vi "GetGrabberPosition.vi"(8 "error in (no error)":errorcluster, 11 "JKI.Robot.SMO.Base.lvclass":refnum<class "JKI.Robot.SMO.Base.lvclass">) -> (0 "error out":errorcluster, 2 "SetGrabberPosition":dbl, 3 "JKI.Robot.SMO.Base.lvclass":refnum<class "JKI.Robot.SMO.Base.lvclass">)   [LabVIEW 2014, in "JKI.Robot.SMO.Base.lvclass"]
doc: "---------------------------------------------------------------\nJKI State Machine Objects™\nhttp://jki.net/state-machine-objects/\nCopyright (C) 2005-2015, JKI <info@jki.net>\nALL RIGHTS RESERVEDJKI State Machine Objects (SMO) 1.0.0.4\nJKI - JKI\nCopyright (c) 2015, JKI"
uses:
  JKI.Robot.SMO.Base.lvclass
panel:
  # "For instructions on how to use the JKI State Machine Objects, examples and video tutorials, visit:\nhttp://jki.net/state-machine-objects/\n\nJKI State Machine Objects™\nhttp://jki.net/state-machine-objects/\nCopyright (C) 2005-2015, JKI <info@jki.net>\nALL RIGHTS RESERVED"
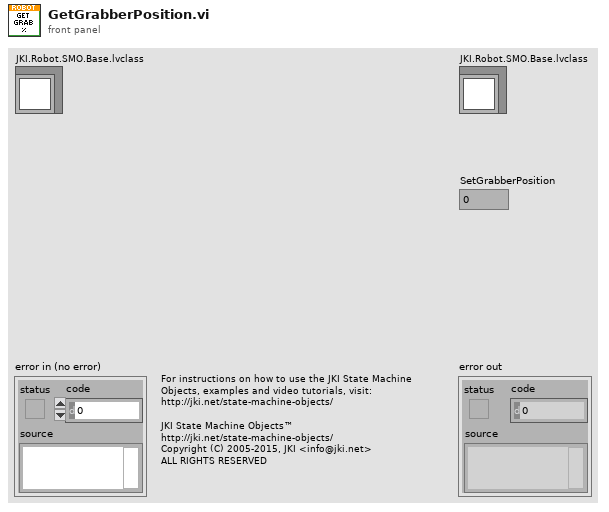
[diagram p1: front panel]
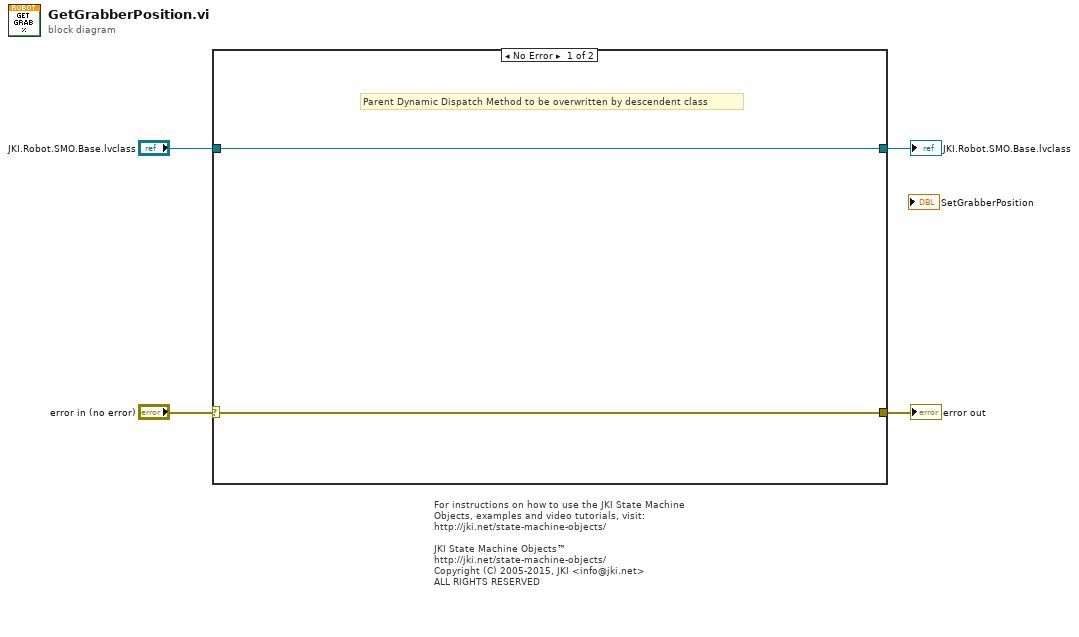
[diagram p0: block diagram]
diagram:
  # "For instructions on how to use the JKI State Machine Objects, examples and video tutorials, visit:\nhttp://jki.net/state-machine-objects/\n\nJKI State Machine Objects™\nhttp://jki.net/state-machine-objects/\nCopyright (C) 2005-2015, JKI <info@jki.net>\nALL RIGHTS RESERVED"
  n1 = case shown="No Error" "error in (no error)" {
    selector: "error in (no error)" -> [w5 w8]
    tunnel: [w5 w8] -> w3
    tunnel: [w6 w7] -> w4
    tunnel: "JKI.Robot.SMO.Base.lvclass" -> [w6 w7]
    frame No Error {
      # "Parent Dynamic Dispatch Method to be overwritten by descendent class"
    }
    frame Error {
    }
  }
  "error out" <- w3
  "JKI.Robot.SMO.Base.lvclass" <- w4
